vi "K2000_config.vi"(1 "Readout_inst_parameters":T1) -> (0 "error out":errorcluster)   [LabVIEW 2013]
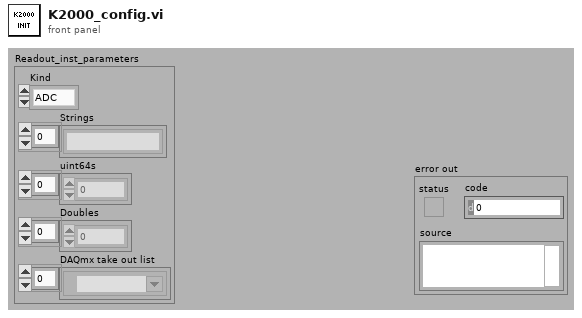
[diagram p1: front panel]
types:
  T1 = cluster{"Kind":enum16{"ADC", "K2000", "34401A", "LeCroy"}, "Strings":string[], "uint64s":u64[], "Doubles":dbl[], "DAQmx take out list":refnum<k21>[]}
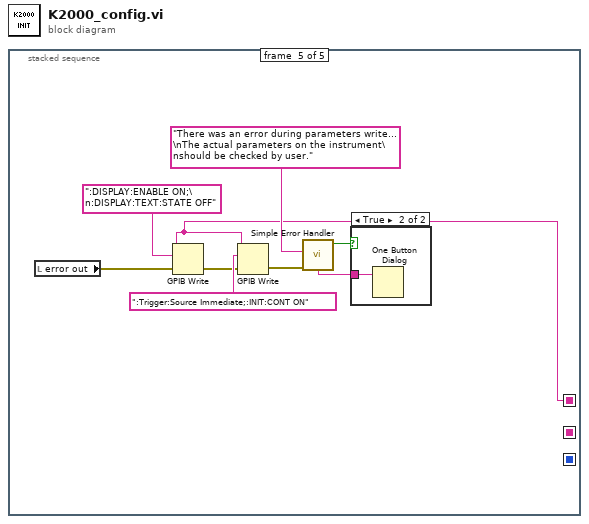
[diagram p0: block diagram]
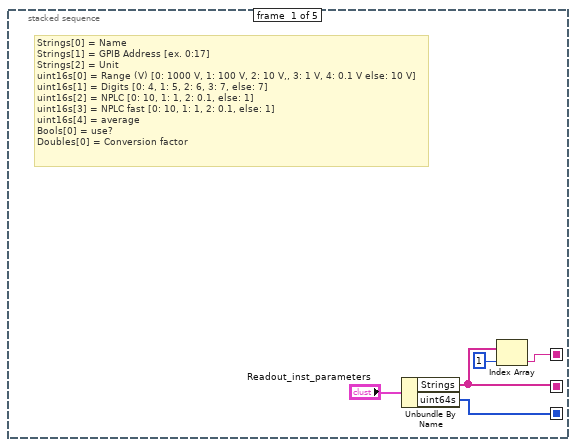
[diagram p2: hidden frame]
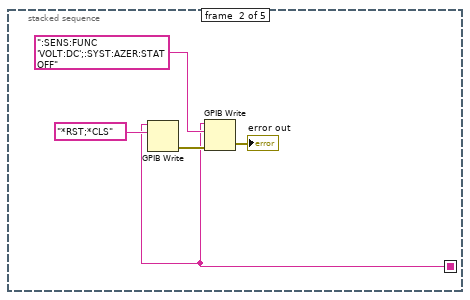
[diagram p3: hidden frame]
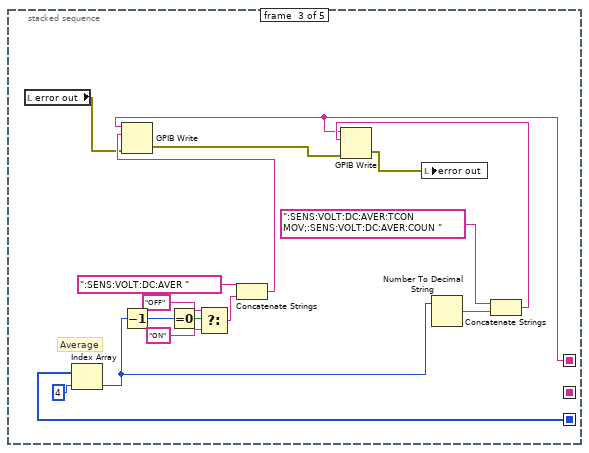
[diagram p4: hidden frame]
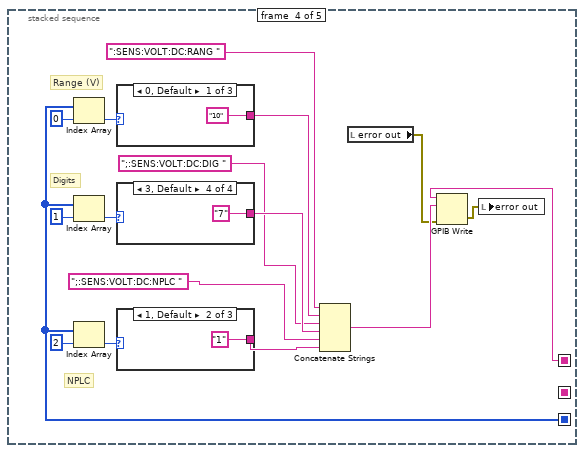
[diagram p5: hidden frame]
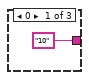
[diagram p6: hidden frame]
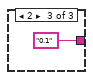
[diagram p7: hidden frame]
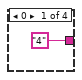
[diagram p8: hidden frame]
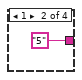
[diagram p9: hidden frame]
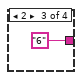
[diagram p10: hidden frame]
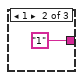
[diagram p11: hidden frame]
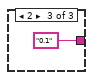
[diagram p12: hidden frame]
diagram:
  n1 = stacked-sequence {
    seq-local: [w2 _ _ _ _] -> [_ _ _ _ _]
    seq-local: [w1 _ _ _ _] -> [_ _ w20 w35 _]
    seq-local: [w3 _ _ _ _] -> [_ w7 w11 w30 w56]
    frame #0 {
      # "Strings[0] = Name\nStrings[1] = GPIB Address [ex. 0:17]\nStrings[2] = Unit\nuint16s[0] = Range (V) [0: 1000 V, 1: 100 V, 2: 10 V,, 3: 1 V, 4: 0.1 V else: 10 V]\nuint16s[1] = Digits [0: 4, 1: 5, 2: 6, 3: 7, else: 7]\nuint16s[2] = NPLC [0: 10, 1: 1, 2: 0.1, else: 1]\nuint16s[3] = NPLC fast [0: 10, 1: 1, 2: 0.1, else: 1]\nuint16s[4] = average\nBools[0] = use?\nDoubles[0] = Conversion factor"
      n2 = Unbundle By Name("Readout_inst_parameters") -> ("Strings"=w2:string[], "uint64s"=w1:u64[])
      n3 = Index Array(array=w2, index=1) -> (element=w3:string)
    }
    frame #1 {
      n4 = GPIB Write(0:w7, 1:"*RST;*CLS" ("data")) -> (6:w10:errorcluster)  [unwired: 1 in, 3 out]
      n5 = GPIB Write(0:w7, 1:":SENS:FUNC 'VOLT:DC';:SYST:AZER:STAT OFF" ("data"), 3:w10) -> (6:→"error out":errorcluster)  [unwired: 3 out]
    }
    frame #2 {
      # "Average"
      n6 = local read "error out"() -> (w18:errorcluster)
      n7 = Index Array(array=w20, index=4) -> (element=w13:u64)
      n8 = Decrement(x=w13) -> (x-1=w26:u64)
      n9 = Equal To 0?(x=w26) -> (x = 0?=w23:bool)
      n10 = Select(t="OFF" ("string"), s=w23, f="ON" ("string")) -> (s? t:f=w27:string)
      n11 = Concatenate Strings(":SENS:VOLT:DC:AVER " ("data"), w27) -> (w19:string)
      n12 = GPIB Write(0:w11, 1:w19, 3:w18) -> (6:w17:errorcluster)  [unwired: 3 out]
      n13 = Number To Decimal String(number=w13) -> (decimal integer string=w15:string)  [unwired: 1 out]
      n14 = Concatenate Strings(":SENS:VOLT:DC:AVER:TCON MOV;:SENS:VOLT:DC:AVER:COUN " ("data"), w15) -> (w12:string)
      n15 = GPIB Write(0:w11, 1:w12, 3:w17) -> (6:w16:errorcluster)  [unwired: 3 out]
      n16 = local write "error out"(w16) -> ()
    }
    frame #3 {
      # "NPLC"
      # "Digits"
      # "Range (V)"
      n17 = Index Array(array=w35, index=0) -> (element=w40:u64)
      n18 = Index Array(array=w35, index=1) -> (element=w42:u64)
      n19 = Index Array(array=w35, index=2) -> (element=w43:u64)
      n20 = case shown="0, Default" w40 {
        tunnel: ["10" "1" "0.1"] -> w41
        frame 0, Default {
        }
        frame 1 {
        }
        frame 2 {
        }
      }
      n21 = case shown="3, Default" w42 {
        tunnel: ["4" ("string") "5" ("string") "6" ("string") "7" ("string")] -> w34
        frame 0 {
        }
        frame 1 {
        }
        frame 2 {
        }
        frame 3, Default {
        }
      }
      n22 = case shown="1, Default" w43 {
        tunnel: ["10" "1" "0.1"] -> w44
        frame 0 {
        }
        frame 1, Default {
        }
        frame 2 {
        }
      }
      n23 = Concatenate Strings(":SENS:VOLT:DC:RANG " ("string"), w41, ";:SENS:VOLT:DC:DIG " ("string"), w34, ";:SENS:VOLT:DC:NPLC " ("string"), w44) -> (w31:string)
      n24 = local read "error out"() -> (w28:errorcluster)
      n25 = GPIB Write(0:w30, 1:w31, 3:w28) -> (6:w29:errorcluster)  [unwired: 3 out]
      n26 = local write "error out"(w29) -> ()
    }
    frame #4 {
      n27 = local read "error out"() -> (w55:errorcluster)
      n28 = GPIB Write(0:w56, 1:":DISPLAY:ENABLE ON;\n:DISPLAY:TEXT:STATE OFF" ("data"), 3:w55) -> (6:w60:errorcluster)  [unwired: 1 in, 2 out]
      n29 = GPIB Write(0:w56, 1:":Trigger:Source Immediate;:INIT:CONT ON" ("data"), 3:w60) -> (6:w62:errorcluster)  [unwired: 1 in, 2 out]
      n30 = call <vilib>:"Simple Error Handler.vi"("error source (\" \")"="There was an error during parameters write...\nThe actual parameters on the instrument\nshould be checked by user." ("error source (\" \")"), "error in (no error)"=w62) -> ("error?"=w58:bool, "message"=w57:string)  [unwired: 1 in, 5 out]
      n31 = case shown="True" w58 {
        tunnel: w57 -> [_ w64]
        frame False {
        }
        frame True {
          n32 = One Button Dialog(message=w64) -> ()  [unwired: 2 out]
        }
      }
    }
  }
